vi "write data type.vi"(8 "error in":errorcluster, 10 "data type":T1, 11 "system tag in":refnum<class "data bus tag description.lvclass">) -> (0 "error out":errorcluster, 3 "system tag out":refnum<class "data bus tag description.lvclass">)   [LabVIEW 2013, in "data bus tag description.lvclass"]
doc: "Write the value of the data type enum in a given tag descriptor."
uses:
  data bus tag description.lvclass
  Data Type.ctl
  data bus tag description.lvclass/data bus tag description.ctl
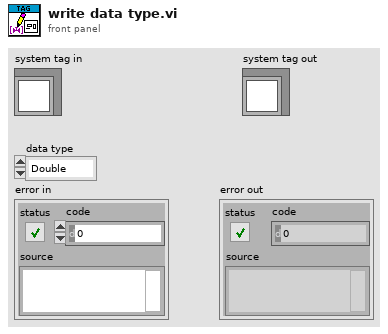
[diagram p1: front panel]
types:
  T1 = typedef "data bus tag description.lvclass/Data Type.ctl" = enum16{"Double", "I64", "Boolean", "Array of Double", "Array of I64", "Variant"}
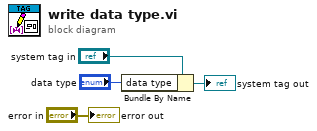
[diagram p0: block diagram]
diagram:
  n1 = Bundle By Name(cluster="system tag in", "data type"="data type") -> (→"system tag out":refnum<class "data bus tag description.lvclass">)
  "error out" <- "error in"
